vi "데이터(2) 저장_위치벡터  txt파일로 저장.vi"(0 "Location":path, 1 "Data2":dbl, 2 "Data1":dbl) -> ()   [LabVIEW 2016]
panel:
  out "Combined Data":string
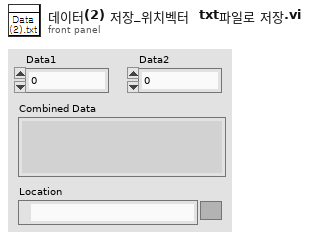
[diagram p1: front panel]
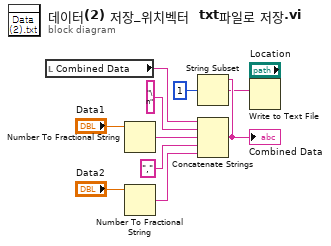
[diagram p0: block diagram]
diagram:
  n1 = local read "Combined Data"() -> (w6:string)
  n2 = Number To Fractional String(number="Data1") -> (F-format string=w11:string)  [unwired: 3 in]
  n3 = Number To Fractional String(number="Data2") -> (F-format string=w10:string)  [unwired: 3 in]
  n4 = Concatenate Strings ("문자열 연결")(w6, "\n" ("문자열"), w11, "," ("문자열"), w10) -> (w2:string)
  "Combined Data" <- w2
  n5 = String Subset(string=w2, offset (0)=1 ("오프셋(0)")) -> (substring=w1:string)  [unwired: 1 in]
  n6 = Write to Text File(file (use dialog)="Location", text=w1) -> ()  [unwired: 2 in, 3 out]
